vi "Evaluate Part 1.vi"() -> ()   [LabVIEW 2020]
uses:
  Map/Maze.lvclass
panel:
  out "Distance":i32
  in  "Input":string=".....\n.S-7.\n.|.|.\n.L-J.\n....."
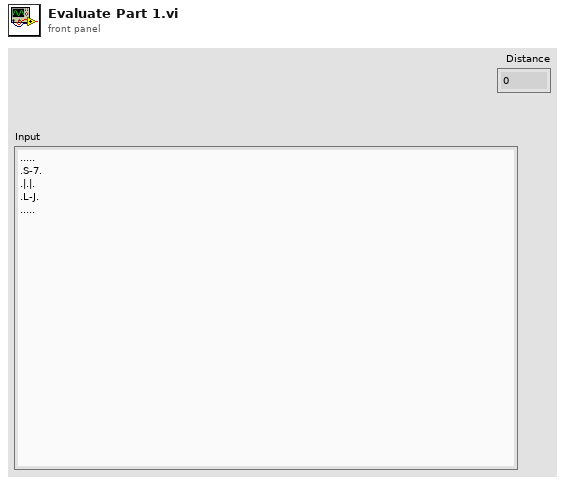
[diagram p1: front panel]
types:
  T1 = typedef "Maze.lvclass/Position.ctl" = cluster{"Row":u64, "Col":u64, "Next Move":enum16{"North", "East", "South", "West", "Halt"}}
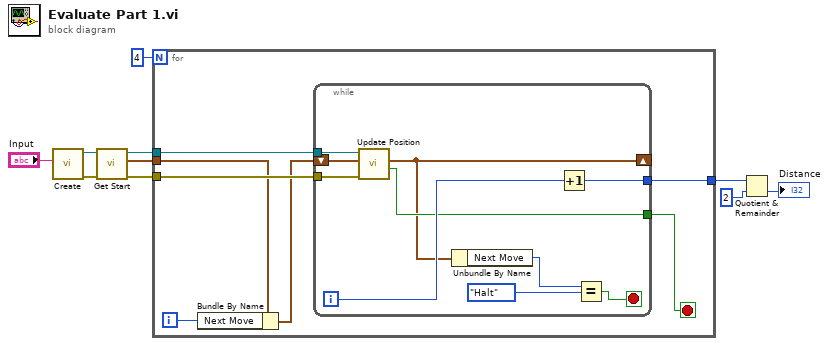
[diagram p0: block diagram]
diagram:
  n1 = call "Create.vi"("Input"="Input") -> ("error out"=w9:errorcluster, "Map"=w10:refnum<class "Maze.lvclass">)  [unwired: 9 in]
  n2 = call "Get Start.vi"("error in (no error)"=w9, "Map in"=w10) -> ("error out"=w7:errorcluster, "Start Vectors"=w5:T1, "Map out"=w8:refnum<class "Maze.lvclass">)  [unwired: 7 in]
  n3 = for {
    N: 4 -> [_]
    tunnel: w8 -> [w17]
    tunnel: w7 -> [w16]
    tunnel: w5 -> [w15]
    tunnel: [w12] -> w3
    i -> [w11]
    stop <- w13 stop-if-true
    n4 = Bundle By Name(cluster=w15, "Next Move"=w11) -> (w14:T1)
    n5 = while {
      tunnel: w17 -> [w27]
      tunnel: w16 -> [w26]
      shift-right: [w21] -> _
      shift-left: w14 -> [w25]
      tunnel: [w22] -> w13
      tunnel: [w18] -> w12
      i -> [w24]
      stop <- w19 stop-if-true
      n6 = call "Update Position.vi"("error in (no error)"=w26, "Current"=w25, "Map In"=w27) -> ("At Start?"=w22:bool, "Next"=w21:T1)  [unwired: 5 in, 2 out]
      n7 = Unbundle By Name(w21) -> ("Next Move"=w20:enum16{"North", "East", "South", "West", "Halt"})
      n8 = Increment(x=w24) -> (x+1=w18:i32)
      n9 = Equal?(x=w20, y=enum16{"North", "East", "South", "West", "Halt"}."Halt") -> (x = y?=w19:bool)
    }
  }
  n10 = Quotient & Remainder(x=w3, y=2) -> (floor(x/y)=→"Distance":i32)  [unwired: 1 out]
